vi "ex2_basic.vi"() -> ()   [LabVIEW 2012]
panel:
  out "error out":errorcluster
  in  "error in (no error)":errorcluster
  in  "stop":bool
  out "Preview Window":picture
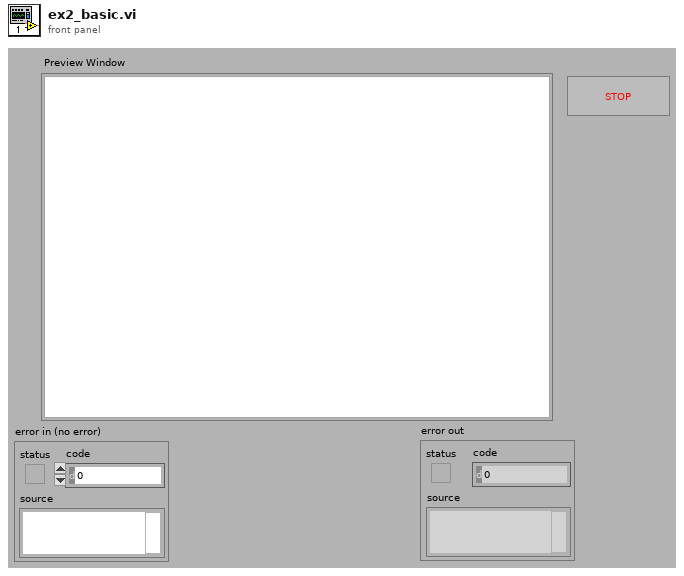
[diagram p1: front panel]
types:
  T1 = typedef "IMAQ Image.ctl" = refnum<image>
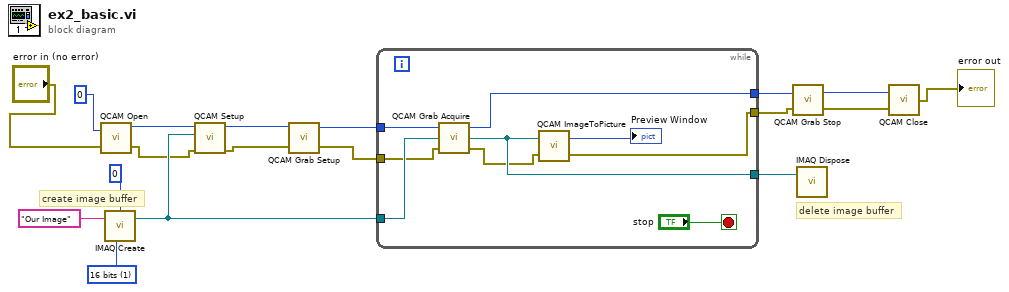
[diagram p0: block diagram]
diagram:
  w18 = u32 1 items=["8 bits", "16 bits"] ("Image Type")
  # "create image buffer"
  # "delete image buffer"
  n1 = call "QCAM Open.vi"("error in (no error)"="error in (no error)", "cameraId"=0) -> ("error out"=w8:errorcluster, "cameraId out"=w13:u32)
  n2 = call "IMAQ Create"("Border Size"=0, "Image Name"="Our Image", "Image Type"=w18) -> ("New Image"=w12:T1)  [unwired: 1 in, 2 out]
  n3 = call "QCAM Setup.vi"("error in (no error)"=w8, "Image"=w12, "cameraId"=w13) -> ("error out"=w7:errorcluster, "cameraId out"=w14:u32)  [unwired: 3 in, 4 out]
  n4 = call "QCAM Grab Setup.vi"("error in (no error)"=w7, "cameraId"=w14) -> ("error out"=w6:errorcluster, "cameraId out"=w17:u32)
  n5 = while {
    tunnel: [w22] -> w10
    tunnel: w12 -> [w23]
    tunnel: w17 -> [w25]
    tunnel: [w26] -> w16
    tunnel: w6 -> [w21]
    tunnel: [w19] -> w3
    stop <- "stop" stop-if-true
    n6 = call "QCAM Grab Acquire.vi"("error in (no error)"=w21, "Image"=w23, "cameraId"=w25) -> ("error out"=w20:errorcluster, "Image Out"=w22:T1, "cameraId out"=w26:u32)
    n7 = call <userlib>:"QCAM ImageToPicture.vi"("error in (no error)"=w20, "Image"=w22) -> ("error out"=w19:errorcluster, "Picture Out"=→"Preview Window":picture)
  }
  n8 = call "QCAM Grab Stop.vi"("error in (no error)"=w3, "cameraId"=w16) -> ("error out"=w2:errorcluster, "cameraId Out"=w11:u32)
  n9 = call "IMAQ Dispose"("Image"=w10) -> ()  [unwired: 2 in, 4 out]
  n10 = call "QCAM Close.vi"("error in (no error)"=w2, "cameraId"=w11) -> ("error out"=→"error out":errorcluster)
